vi "save prueba.vi"(8 "error in (no error)":errorcluster, 11 "Nombre de la Prueba":string) -> (0 "error out":errorcluster)   [LabVIEW 2020, in "Settings.lvlib"]
uses:
  Settings.lvlib
  <vilib>/drjdpowell/SQLite Library/SQL Connection/Open (path).vi
  <vilib>/drjdpowell/SQLite Library/SQL Connection/Open (string).vi
  <vilib>/AdvancedString/Path To Command Line String.vi
  <vilib>/drjdpowell/SQLite Library/SQL Connection/Execute SQL (No results).vi
  <vilib>/drjdpowell/SQLite Library/SQL Connection/Connection.lvclass
  <vilib>/drjdpowell/SQLite Library/SQLite.lvlib
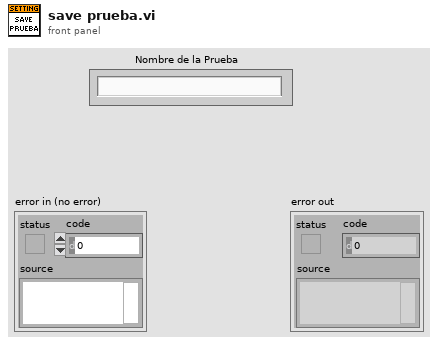
[diagram p1: front panel]
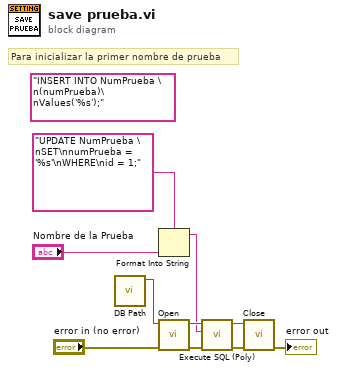
[diagram p0: block diagram]
diagram:
  (unwired) "INSERT INTO NumPrueba \n(numPrueba)\nValues('%s');"
  # "Para inicializar la primer nombre de prueba"
  n1 = call "DB Path.vi"() -> ("DB path"=w4:path)  [unwired: 11 in]
  n2 = Format Into String(format string="UPDATE NumPrueba \nSET\nnumPrueba = '%s'\nWHERE\nid = 1;", "Nombre de la Prueba") -> (resulting string=w2:string)  [unwired: 2 in, 1 out]
  n3 = call-poly <vilib>:"Open.vi"("error in (no error)"="error in (no error)", "db file"=w4) -> ("error out"=w10:errorcluster, "SQLite Connection"=w9:refnum<class "Connection.lvclass">)  [unwired: 8 in]
  n4 = call-poly <vilib>:"Execute SQL (Poly).vi"("error in (no error)"=w10, "SQL"=w2, "SQLite Connection in"=w9) -> ("error out"=w7:errorcluster, "SQLite Connection"=w8:refnum<class "Connection.lvclass">)  [unwired: 7 in]
  n5 = call-dynamic "Close.vi"("error in (no error)"=w7, "SQLite Connection in"=w8) -> ("error out"=→"error out":errorcluster)  [unwired: 9 in]
